vi "Acquisition Increment.vi"(8 "error in (no error)":errorcluster, 11 "Top Level in":refnum<class "Top Level.lvclass">) -> (0 "error out":errorcluster, 3 "Top Level out":refnum<class "Top Level.lvclass">)   [LabVIEW 2021, in "Top Level.lvlib" / "Top Level.lvclass"]
uses:
  Top Level.lvclass
  Top Level.lvclass/Top Level.ctl
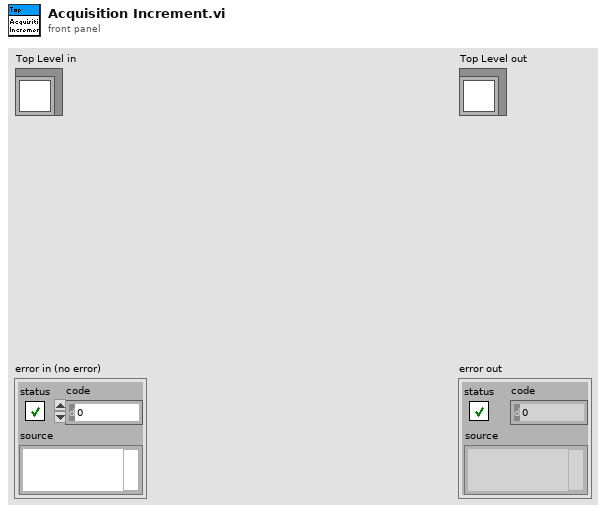
[diagram p1: front panel]
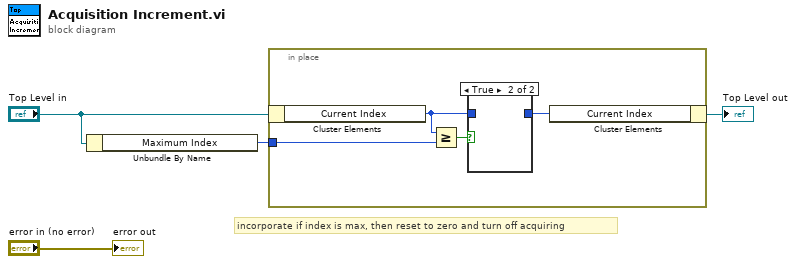
[diagram p0: block diagram]
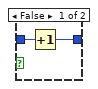
[diagram p2: hidden frame]
diagram:
  # "incorporate if index is max, then reset to zero and turn off acquiring"
  n1 = Unbundle By Name("Top Level in") -> ("Maximum Index"=w3:i32)
  n2 = in-place {
    in-place-border: w3 -> [w5]
    n3 = in-place-cluster #1("Top Level in") -> ("Current Index"=w6:i32)
    n4 = Greater Or Equal?(x=w6, y=w5) -> (x >= y?=w8:bool)
    n5 = case shown="True" w8 {
      tunnel: w6 -> [w10 _]
      tunnel: [w9 _] -> w7
      frame False {
        n6 = Increment(x=w10) -> (x+1=w9:i32)
      }
      frame True {
      }
    }
    n7 = in-place-cluster #1("Current Index"=w7) -> (→"Top Level out":refnum<class "Top Level.lvclass">)
  }
  "error out" <- "error in (no error)"
